vi "read (CryoCon).vi"(2 "error in (no error)":errorcluster, 3 "VISA resource name":refnum<visa-resource-name>) -> (0 "error out":errorcluster, 1 "read buffer":string)   [LabVIEW 2011]
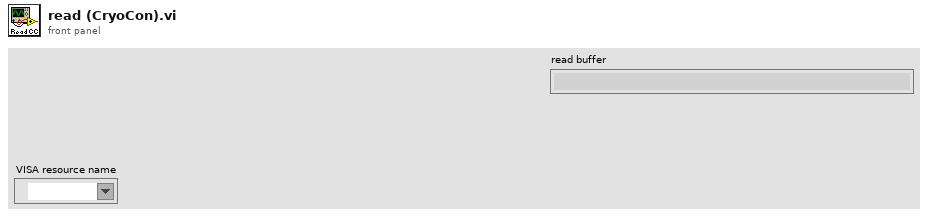
[diagram p1: front panel]
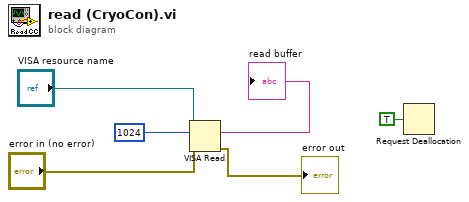
[diagram p0: block diagram]
diagram:
  n1 = VISA Read(VISA resource name="VISA resource name", byte count=u32 1024, error in (no error)="error in (no error)") -> (read buffer=→"read buffer":string, error out=→"error out":errorcluster)  [unwired: 2 out]
  n2 = Request Deallocation(TRUE ("flag")) -> ()
